vi "RVHR - Define RunTime Menu.vi"(8 "error in (no error)":errorcluster, 9 "UI Information.Language":T1=enum."Chinese", 10 "Language Config Cluster Out":T2={"Home"="", "Test Setup"="", "Run Test"="", "Configure"="", "Hardware Viewer"="", "Review Test"="", "Report"="", "Exit"="", "Device Connected?"="", "Test in Progress?"="", "Simulate?"="", "Device Type 1"="", "Device Type 2"="", "Device Type 3"="", "Device Type 4"="", "Device Type 5"="Bi-Corrugation Analysis Trolley", "Device Type 6"="Bi-Corrugation Analysis Trolley", "Device Type 7"="Bi-Corrugation Analysis Trolley", "Software Version"="", "Support"="", "Operator"="", "Test Description"="", "Line"="", "Test Folder Path"="", "Test Folder Path RCA"="", "Start Position"="", "Sensor Position"="", "Sensor A Position"="", "Sensor B Position"="", "Visible Chart Distance"="", "Rail Side"="", "Rail A Side"="", "Distance Direction"="", "Start"="", "Distance Travelled"="", "Current Position"="", "Stop Test"="", "Pause Test"="", "Displacement"="", "Position"="", "Sensor Calibration"="", "Sensor A Calibration"="", "Sensor B Calibration"="", "Encoder Spacing"="", "Sampling Distance"="", "Tacho Pulses/Rev"="", "Wheel Diameter"="", "Sampling Distances"=[], "Distance Unit"="", "Distance Units"=[], "Swap Direction"="", "Language"="", "Device Resolution"="", "Device Resolutions"=[], "Detect Change in Direction"="", "Save Config"="", "Encoder Data"="", "Sensor Data"="", "Sensor A Data"="", "Sensor B Data"="", "Voltage"="", "Time (m:s)"="", "Unit mm/s/V"="", "Unit mm"="", "Unit km"="", "Unit m"="", "Start Test Message"="", "Stop Test Message"="", "Exit Message"="", "File Exists Message"="", "File Path Invalid Message"="", "Combine Error"="", "Combine Success"="", "Roller Comp Error"="", "Test Folder Path (Live)"="", "Folder Error"="", "Enc Count"="", "Run Start"="", "Run End"="", "Date"="", "Train"="", "Location"="", "Notes"="", "Heading_1"="", "Heading_2"="", "Left Rail"="", "Right Rail"="", "Left Exclusions"="", "Right Exclusions"="", "Settings"="", "Wavelength Ranges"="", "Y-Axis Limits"="", "Exc Limits"="", "Other Settings"="", "Distance/Page"="", "Distance/Pages"=[], "Gridlines"="", "Report Tolerance"="", "Manual Cut"="", "Plot Colour"="", "Plot Colours"=[], "EN Standard"="", "RiL Standard"="", "Custom Standard"="", "Resolution"="", "Resolutions"=[], "Exceedence Header"="", "Distance (km)"="", "Left (%)"="", "Right (%)"="", "Page"="", "Align"="", "Main"="", "Comparison"="", "Offset"="", "From"="", "To"="", "Of"="Distance in:", "File"="", "Load New"="", "Load Comparison"="", "Discard Comparison"="", "Print Current Page"="", "Print All Pages"="", "Print Exceedence Report"="", "Plot Main"="", "No Comparison Data to Align"="Distance in:", "Run Load Error"="Distance in:", "Report Load Error"="Distance in:", "Cut"="Distance in:", "Remove"="Distance in:", "Config Settings Unsaved"="Distance in:", "Acquisition Paused"="Distance in:", "Please Select One Option Below"="Distance in:", "RCA is Now Stationary"="Distance in:", "Reporting Setting"="Distance in:", "Main Abbreviated"="Distance in:", "Comparison Abbreviated"="Distance in:", "Exceedence Abbreviated"="Distance in:", "Align Comparison"="Distance in:", "Rail Corrugation Analyser Reporting"="Distance in:", "Show Exc. % in Graph"="Distance in:", "Evaluate Sections <100m"="Distance in:", "Evaluate Sections <0.062mile"="Distance in:", "Section Too Short for Evaluation"="Distance in:", "Language Change Prompt"="Distance in:", "Show All"="Distance in:", "Sections_km"="Distance in:", "Sections_mi"="Distance in:", "Vision"="Distance in:", "Vision Report"="Distance in:", "Vision Display"="Distance in:", "Vision Displays"=["Kilometres", "miles & chains", "metres", "stations", "miles"], "Save Images"="Distance in:", "Image Frequency"="Distance in:", "Section"="Distance in:", "Brightness"="Distance in:", "Contrast"="Distance in:", "Shadow"="Distance in:", "Sharpened"="Distance in:", "Apply to all Images"="Distance in:", "Reset"="Distance in:", "Are you sure"="Distance in:", "Image Processing"="Distance in:", "Save Video"="Distance in:", "Image Offset"="Distance in:", "Camera Mode"="Distance in:", "Camera Modes"=["Kilometres", "miles & chains", "metres", "stations", "miles"], "Copy Page"="Distance in:", "Copy Graphs"="Distance in:", "Camera Mode Change Prompt"="Distance in:", "Camera_1 Missing"="Distance in:", "Camera_2 Missing"="Distance in:", "Cameras Missing"="Distance in:", "Camera Setup"="Distance in:", "Camera_1 Connection Error"="Distance in:", "Camera_2 Connection Error"="Distance in:", "Cameras Connection Error"="Distance in:", "No GPS"="Distance in:", "No Signal"="Distance in:", "Camera_1 Connected"="Distance in:", "Camera_1 Not Connected"="Distance in:", "Camera_2 Connected"="Distance in:", "Camera_2 Not Connected"="Distance in:", "Start Position at 0m?"="Distance in:", "Continue"="Distance in:", "New Test, Same Direction"="Distance in:", "New Test, Opposite Direction"="Distance in:", "Stop and Save"="Distance in:", "Live Corrug Estimate"="Distance in:", "Wavelength Corrug"="Distance in:", "Distance Corrug "="Distance in:", "Update Corrug"="Distance in:", "Company"="Distance in:", "Ref Profile "="Distance in:", "Company_Report"="Distance in:", "Ref Profile_Report"="Distance in:", "Heading_1_RVHR"="Distance in:", "Heading_2_RVHR"="Distance in:", "Remove Feature"="Distance in:", "Feature Type"="Sampling Distance:", "Feature Types"=["1mm", "2mm"], "AI Not Ready"="Sampling Distance:"}, 11 "Menu in":refnum<k9>) -> (0 "error out":errorcluster)   [LabVIEW 2024]
uses:
  Controls/Language Vision Text Cluster.ctl
  Controls/Language.ctl
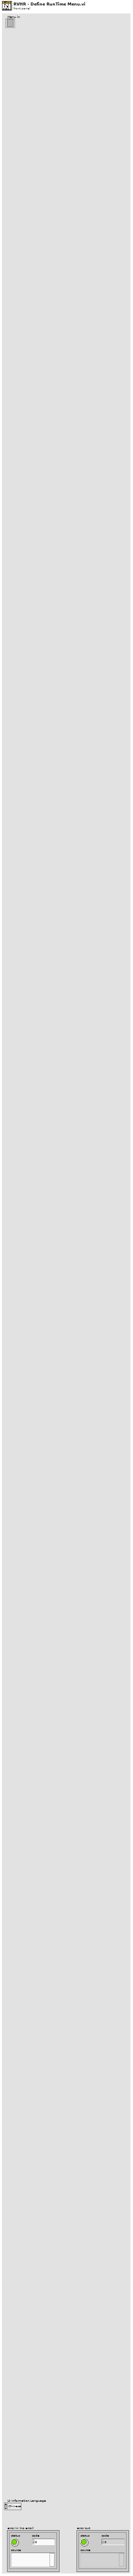
[diagram p1: front panel]
types:
  T1 = typedef "Language.ctl" = enum16{"English", "Chinese", "German"}
  T2 = typedef "Language Vision Text Cluster.ctl" = cluster{"Home":string, "Test Setup":string, "Run Test":string, "Configure":string, "Hardware Viewer":string, "Review Test":string, "Report":string, "Exit":string, "Device Connected?":string, "Test in Progress?":string, "Simulate?":string, "Device Type 1":string, "Device Type 2":string, "Device Type 3":string, "Device Type 4":string, "Device Type 5":string, "Device Type 6":string, "Device Type 7":string, "Software Version":string, "Support":string, "Operator":string, "Test Description":string, "Line":string, "Test Folder Path":string, "Test Folder Path RCA":string, "Start Position":string, "Sensor Position":string, "Sensor A Position":string, "Sensor B Position":string, "Visible Chart Distance":string, "Rail Side":string, "Rail A Side":string, "Distance Direction":string, "Start":string, "Distance Travelled":string, "Current Position":string, "Stop Test":string, "Pause Test":string, "Displacement":string, "Position":string, "Sensor Calibration":string, "Sensor A Calibration":string, "Sensor B Calibration":string, "Encoder Spacing":string, "Sampling Distance":string, "Tacho Pulses/Rev":string, "Wheel Diameter":string, "Sampling Distances":string[], "Distance Unit":string, "Distance Units":string[], "Swap Direction":string, "Language":string, "Device Resolution":string, "Device Resolutions":string[], "Detect Change in Direction":string, "Save Config":string, "Encoder Data":string, "Sensor Data":string, "Sensor A Data":string, "Sensor B Data":string, "Voltage":string, "Time (m:s)":string, "Unit mm/s/V":string, "Unit mm":string, "Unit km":string, "Unit m":string, "Start Test Message":string, "Stop Test Message":string, "Exit Message":string, "File Exists Message":string, "File Path Invalid Message":string, "Combine Error":string, "Combine Success":string, "Roller Comp Error":string, "Test Folder Path (Live)":string, "Folder Error":string, "Enc Count":string, "Run Start":string, "Run End":string, "Date":string, "Train":string, "Location":string, "Notes":string, "Heading_1":string, "Heading_2":string, "Left Rail":string, "Right Rail":string, "Left Exclusions":string, "Right Exclusions":string, "Settings":string, "Wavelength Ranges":string, "Y-Axis Limits":string, "Exc Limits":string, "Other Settings":string, "Distance/Page":string, "Distance/Pages":string[], "Gridlines":string, "Report Tolerance":string, "Manual Cut":string, "Plot Colour":string, "Plot Colours":string[], "EN Standard":string, "RiL Standard":string, "Custom Standard":string, "Resolution":string, "Resolutions":string[], "Exceedence Header":string, "Distance (km)":string, "Left (%)":string, "Right (%)":string, "Page":string, "Align":string, "Main":string, "Comparison":string, "Offset":string, "From":string, "To":string, "Of":string, "File":string, "Load New":string, "Load Comparison":string, "Discard Comparison":string, "Print Current Page":string, "Print All Pages":string, "Print Exceedence Report":string, "Plot Main":string, "No Comparison Data to Align":string, "Run Load Error":string, "Report Load Error":string, "Cut":string, "Remove":string, "Config Settings Unsaved":string, "Acquisition Paused":string, "Please Select One Option Below":string, "RCA is Now Stationary":string, "Reporting Setting":string, "Main Abbreviated":string, "Comparison Abbreviated":string, "Exceedence Abbreviated":string, "Align Comparison":string, "Rail Corrugation Analyser Reporting":string, "Show Exc. % in Graph":string, "Evaluate Sections <100m":string, "Evaluate Sections <0.062mile":string, "Section Too Short for Evaluation":string, "Language Change Prompt":string, "Show All":string, "Sections_km":string, "Sections_mi":string, "Vision":string, "Vision Report":string, "Vision Display":string, "Vision Displays":string[], "Save Images":string, "Image Frequency":string, "Section":string, "Brightness":string, "Contrast":string, "Shadow":string, "Sharpened":string, "Apply to all Images":string, "Reset":string, "Are you sure":string, "Image Processing":string, "Save Video":string, "Image Offset":string, "Camera Mode":string, "Camera Modes":string[], "Copy Page":string, "Copy Graphs":string, "Camera Mode Change Prompt":string, "Camera_1 Missing":string, "Camera_2 Missing":string, "Cameras Missing":string, "Camera Setup":string, "Camera_1 Connection Error":string, "Camera_2 Connection Error":string, "Cameras Connection Error":string, "No GPS":string, "No Signal":string, "Camera_1 Connected":string, "Camera_1 Not Connected":string, "Camera_2 Connected":string, "Camera_2 Not Connected":string, "Start Position at 0m?":string, "Continue":string, "New Test, Same Direction":string, "New Test, Opposite Direction":string, "Stop and Save":string, "Live Corrug Estimate":string, "Wavelength Corrug":string, "Distance Corrug ":string, "Update Corrug":string, "Company":string, "Ref Profile ":string, "Company_Report":string, "Ref Profile_Report":string, "Heading_1_RVHR":string, "Heading_2_RVHR":string, "Remove Feature":string, "Feature Type":string, "Feature Types":string[], "AI Not Ready":string}
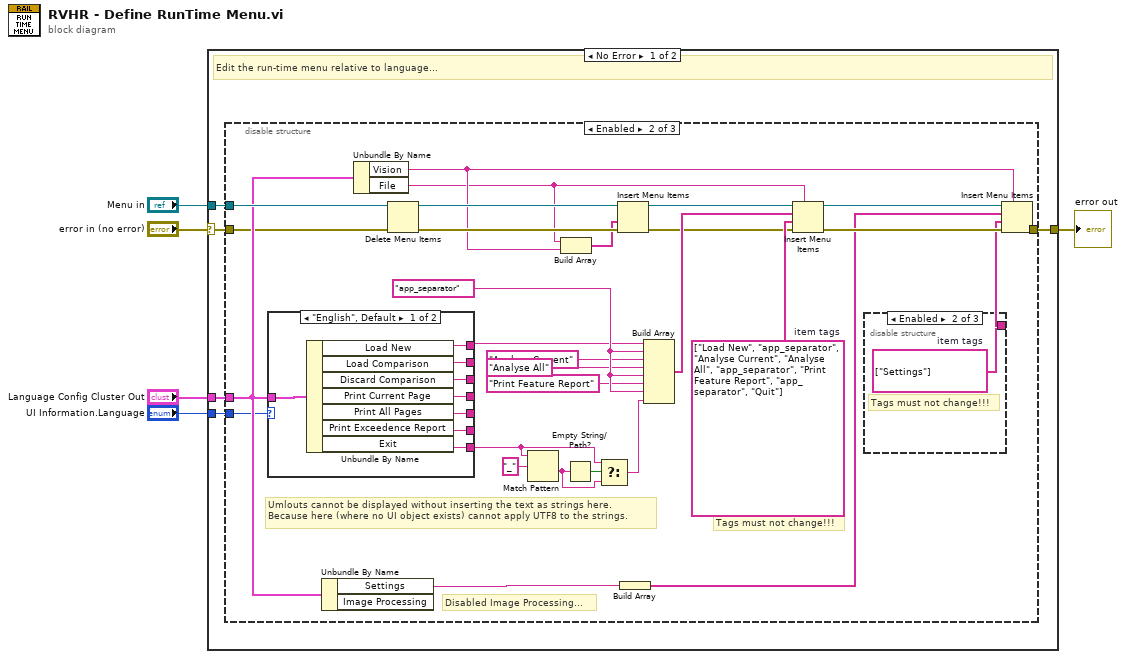
[diagram p0: block diagram]
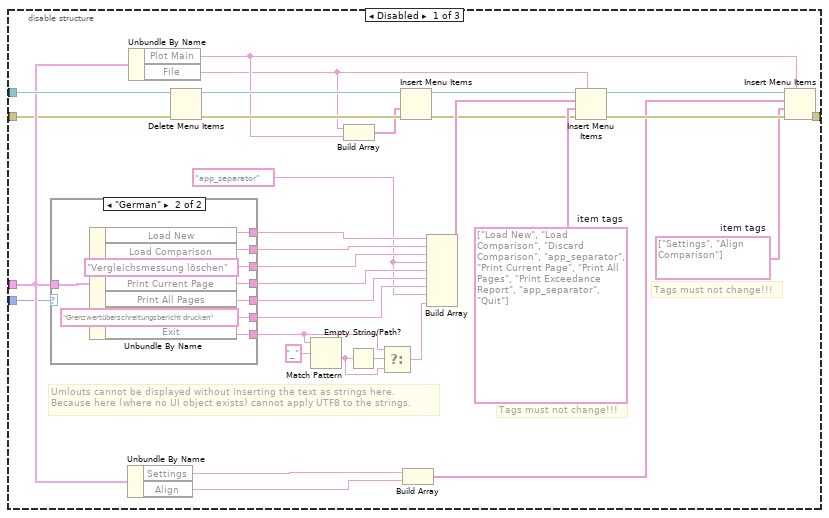
[diagram p2: hidden frame]
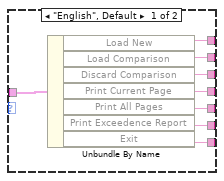
[diagram p3: hidden frame]
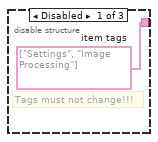
[diagram p4: hidden frame]
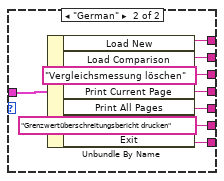
[diagram p6: hidden frame]
diagram:
  n1 = case shown="No Error" "error in (no error)" {
    selector: "error in (no error)" -> [w8 w106]
    tunnel: "Menu in" -> [w10 _]
    tunnel: "Language Config Cluster Out" -> [w9 _]
    tunnel: [w7 w106] -> w5
    tunnel: "UI Information.Language" -> [w6 _]
    frame No Error {
      # "Edit the run-time menu relative to language..."
      n2 = disable-structure shown="Enabled" {
        disable-tunnel: w10 -> [w41 w86 _]
        disable-tunnel: w9 -> [w27 w80 _]
        disable-tunnel: w8 -> [w18 w71 _]
        disable-tunnel: [w17 w70 _] -> w7
        disable-tunnel: w6 -> [w11 w64 _]
        frame Disabled {
          w31 = "app_separator"
          w38 = string[] ["Settings", "Align Comparison"]  # item tags
          w39 = string[] ["Load New", "Load Comparison", "Discard Comparison", "app_separator", "Print Current Page", "Print All Pages", "Print Exceedance Report", "app_separator", "Quit"]  # item tags
          # "Umlouts cannot be displayed without inserting the text as strings here.\nBecause here (where no UI object exists) cannot apply UTF8 to the strings."
          # "Tags must not change!!!"
          # "Tags must not change!!!"
          n3 = case shown="\"German\"" w11 {
            tunnel: [w50 w58] -> w37
            tunnel: [w49 w57] -> w36
            tunnel: [w48 "Vergleichsmessung löschen" ("Discard Comparison")] -> w35
            tunnel: [w47 w56] -> w34
            tunnel: [w46 w55] -> w33
            tunnel: [w45 "Grenzwertüberschreitungsbericht drucken" ("Print Exceedence Report")] -> w32
            tunnel: w27 -> [w44 w54]
            tunnel: [w43 w53] -> w14
            frame "English", Default {
              n4 = Unbundle By Name(w44) -> ("Load New"=w50:string, "Load Comparison"=w49:string, "Discard Comparison"=w48:string, "Print Current Page"=w47:string, "Print All Pages"=w46:string, "Print Exceedence Report"=w45:string, "Exit"=w43:string)
            }
            frame "German" {
              n5 = Unbundle By Name(w54) -> ("Load New"=w58:string, "Load Comparison"=w57:string, "Print Current Page"=w56:string, "Print All Pages"=w55:string, "Exit"=w53:string)  [unwired: 2 out]
            }
          }
          n6 = Unbundle By Name(w27) -> ("Settings"=w28:string, "Align"=w29:string)
          n7 = Unbundle By Name(w27) -> ("Plot Main"=w21:string, "File"=w20:string)
          n8 = Delete Menu Items(6:w18, 9:w41) -> (0:w24:errorcluster, 3:w25:refnum<k9>)  [unwired: 2 in]
          n9 = Match Pattern(string=w14, regular expression="_") -> (after substring=w12:string)  [unwired: 1 in, 3 out]
          n10 = Build Array(w20, w21) -> (w19:string[])
          n11 = Empty String/Path?(string/path=w12) -> (empty?=w15:bool)
          n12 = Select(t=w14, s=w15, f=w12) -> (s? t:f=w13:string)
          n13 = Insert Menu Items(6:w24, 7:w19, 9:w25) -> (0:w23:errorcluster, 3:w22:refnum<k9>)  [unwired: 3 in, 1 out]
          n14 = Build Array(w28, w29) -> (w26:string[])
          n15 = Build Array(w37, w36, w35, w31, w34, w33, w32, w31, w13) -> (w30:string[])
          n16 = Insert Menu Items(5:w20, 6:w23, 7:w39, 8:w30, 9:w22) -> (0:w40:errorcluster, 3:w42:refnum<k9>)  [unwired: 1 in, 1 out]
          n17 = Insert Menu Items(5:w21, 6:w40, 7:w38, 8:w26, 9:w42) -> (0:w17:errorcluster)  [unwired: 1 in, 2 out]
        }
        frame Enabled {
          w63 = "app_separator"
          w84 = string[] ["Load New", "app_separator", "Analyse Current", "Analyse All", "app_separator", "Print Feature Report", "app_separator", "Quit"]  # item tags
          # "Disabled Image Processing..."
          # "Umlouts cannot be displayed without inserting the text as strings here.\nBecause here (where no UI object exists) cannot apply UTF8 to the strings."
          # "Tags must not change!!!"
          n18 = case shown="\"English\", Default" w64 {
            tunnel: [w97 w105] -> w62
            tunnel: [w96 w104] -> _
            tunnel: [w95 "Vergleichsmessung löschen" ("Discard Comparison")] -> _
            tunnel: [w94 w103] -> _
            tunnel: [w93 w102] -> _
            tunnel: [w92 "Grenzwertüberschreitungsbericht drucken" ("Print Exceedence Report")] -> _
            tunnel: w80 -> [w91 w101]
            tunnel: [w90 w100] -> w67
            frame "English", Default {
              n19 = Unbundle By Name(w91) -> ("Load New"=w97:string, "Load Comparison"=w96:string, "Discard Comparison"=w95:string, "Print Current Page"=w94:string, "Print All Pages"=w93:string, "Print Exceedence Report"=w92:string, "Exit"=w90:string)
            }
            frame "German" {
              n20 = Unbundle By Name(w101) -> ("Load New"=w105:string, "Load Comparison"=w104:string, "Print Current Page"=w103:string, "Print All Pages"=w102:string, "Exit"=w100:string)  [unwired: 2 out]
            }
          }
          n21 = Unbundle By Name(w80) -> ("Settings"=w81:string)  [unwired: 1 out]
          n22 = Unbundle By Name(w80) -> ("Vision"=w74:string, "File"=w73:string)
          n23 = Delete Menu Items(6:w71, 9:w86) -> (0:w77:errorcluster, 3:w78:refnum<k9>)  [unwired: 2 in]
          n24 = Match Pattern(string=w67, regular expression="_") -> (after substring=w65:string)  [unwired: 1 in, 3 out]
          n25 = Build Array(w73, w74) -> (w72:string[])
          n26 = Empty String/Path?(string/path=w65) -> (empty?=w68:bool)
          n27 = Select(t=w67, s=w68, f=w65) -> (s? t:f=w66:string)
          n28 = Insert Menu Items(6:w77, 7:w72, 9:w78) -> (0:w76:errorcluster, 3:w75:refnum<k9>)  [unwired: 3 in, 1 out]
          n29 = Build Array(w81) -> (w79:string[])
          n30 = Build Array(w62, w63, "Analyse Current" ("element"), "Analyse All" ("element"), w63, "Print Feature Report" ("element"), w63, w66) -> (w82:string[])
          n31 = Insert Menu Items(5:w73, 6:w76, 7:w84, 8:w82, 9:w75) -> (0:w85:errorcluster, 3:w87:refnum<k9>)  [unwired: 1 in, 1 out]
          n32 = disable-structure shown="Enabled" {
            disable-tunnel: [w88 w89 _] -> w83
            frame Disabled {
              w88 = string[] ["Settings", "Image Processing"]  # item tags
              # "Tags must not change!!!"
            }
            frame Enabled {
              w89 = string[] ["Settings"]  # item tags
              # "Tags must not change!!!"
            }
            frame Disabled {
            }
          }
          n33 = Insert Menu Items(5:w74, 6:w85, 7:w83, 8:w79, 9:w87) -> (0:w70:errorcluster)  [unwired: 1 in, 2 out]
        }
        frame Disabled {
        }
      }
    }
    frame Error {
    }
  }
  "error out" <- w5
